vi "overlay_grid.vi"(3 "no of grid lines":i32(slide)=2 min=0 step=1 scale=2.0..20.0, 4 "Color (red)":u32(colorbox)=16711680, 5 "Image In":T1) -> (2 "Image Out":T1)   [LabVIEW 2017]
doc: "SciScan 1.2 160622"
uses:
  <vilib>/vision/Image Controls.llb/IMAQ Image.ctl
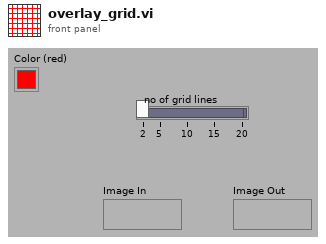
[diagram p1: front panel]
types:
  T1 = typedef "IMAQ Image.ctl" = refnum<image>
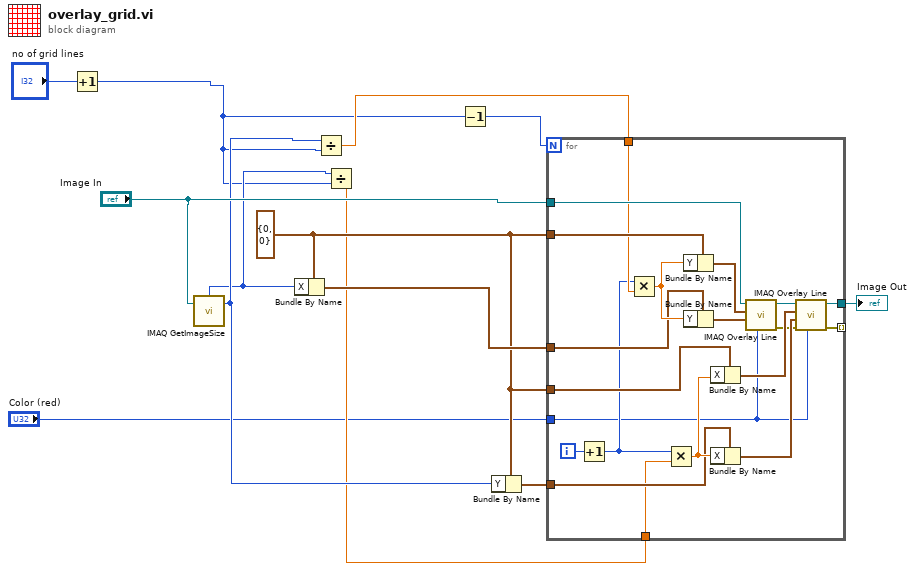
[diagram p0: block diagram]
diagram:
  w9 = cluster{"X":i32, "Y":i32} {"X"=0, "Y"=0} ("Start Point")
  n1 = Increment(x="no of grid lines") -> (x+1=w2:i32)
  n2 = call "IMAQ GetImageSize"("Image"="Image In") -> ("Y Resolution"=w8:i32, "X Resolution"=w7:i32)  [unwired: 3 in, 1 out]
  n3 = Bundle By Name(cluster=w9, "X"=w7) -> (w11:cluster{"X":i32, "Y":i32})
  n4 = Divide(x=w8, y=w2) -> (x/y=w4:dbl)
  n5 = Divide(x=w7, y=w2) -> (x/y=w5:dbl)
  n6 = Decrement(x=w2) -> (x-1=w3:i32)
  n7 = Bundle By Name(cluster=w9, "Y"=w8) -> (w10:cluster{"X":i32, "Y":i32})
  n8 = for {
    N: w3 -> [_]
    tunnel: "Image In" -> [w33]
    tunnel: [w29] -> w13
    tunnel: w9 -> [w23]
    tunnel: w9 -> [w22]
    tunnel: w11 -> [w21]
    tunnel: w10 -> [w20]
    tunnel: w4 -> [w19]
    tunnel: w5 -> [w18]
    tunnel: [w16] -> _ mode=indexing
    tunnel: "Color (red)" -> [w14]
    i -> [w25]
    n9 = Increment(x=w25) -> (x+1=w15:i32)
    n10 = Multiply(x=w15, y=w19) -> (x*y=w26:dbl)
    n11 = Multiply(x=w15, y=w18) -> (x*y=w24:dbl)
    n12 = Bundle By Name(cluster=w23, "Y"=w26) -> (w32:cluster{"X":i32, "Y":i32})
    n13 = Bundle By Name(cluster=w21, "Y"=w26) -> (w31:cluster{"X":i32, "Y":i32})
    n14 = Bundle By Name(cluster=w22, "X"=w24) -> (w28:cluster{"X":i32, "Y":i32})
    n15 = Bundle By Name(cluster=w20, "X"=w24) -> (w27:cluster{"X":i32, "Y":i32})
    n16 = call "IMAQ Overlay Line"("Color"=w14, "End Point"=w31, "Start Point"=w32, "Image"=w33) -> ("error out"=w17:errorcluster, "Image Out"=w30:T1)  [unwired: 6 in]
    n17 = call "IMAQ Overlay Line"("Color"=w14, "error in (no error)"=w17, "End Point"=w27, "Start Point"=w28, "Image"=w30) -> ("error out"=w16:errorcluster, "Image Out"=w29:T1)  [unwired: 5 in]
  }
  "Image Out" <- w13
